vi "Filter and Data Scaling backup (62611) temp.vi"(0 "Offset Data":string[](array[string]), 5 "Slope Data":string[](array[string]), 7 "Filter Data":string[](array[string]), 9 "Vin":dbl[](array[numeric]), 11 "error in":errorcluster, 12 "Allow Zero?":string[](array[string])) -> (4 "Vout":string[](array[string]), 6 "Offset Data":string[](array[string]), 8 "ScaledOut":string[](array[string]), 10 "ScaledOut":dbl[](array[numeric]), 14 "Allow Zero?":string[](array[string]), 15 "error out":errorcluster)   [LabVIEW 2018]
uses:
  Counters.vi
  <vilib>/ptbypt/NI_PtbyPt.lvlib
panel:
  out "k":dbl
  out "fdelta":dbl
  out "fratio":dbl
  out "dp":dbl
  out "Numeric":i32
  # "32-51= FM1 GPM Data Point 1-20"
  # "32-51= FM1 Data Point # 1-20"
  # "32-51 = FM1 K Factor 1-20"
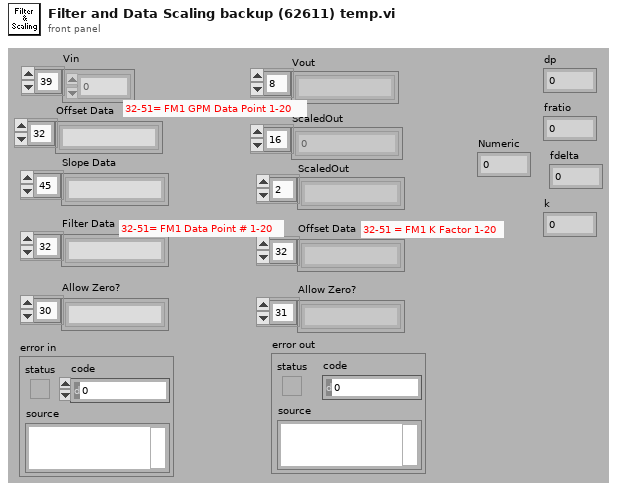
[diagram p1: front panel]
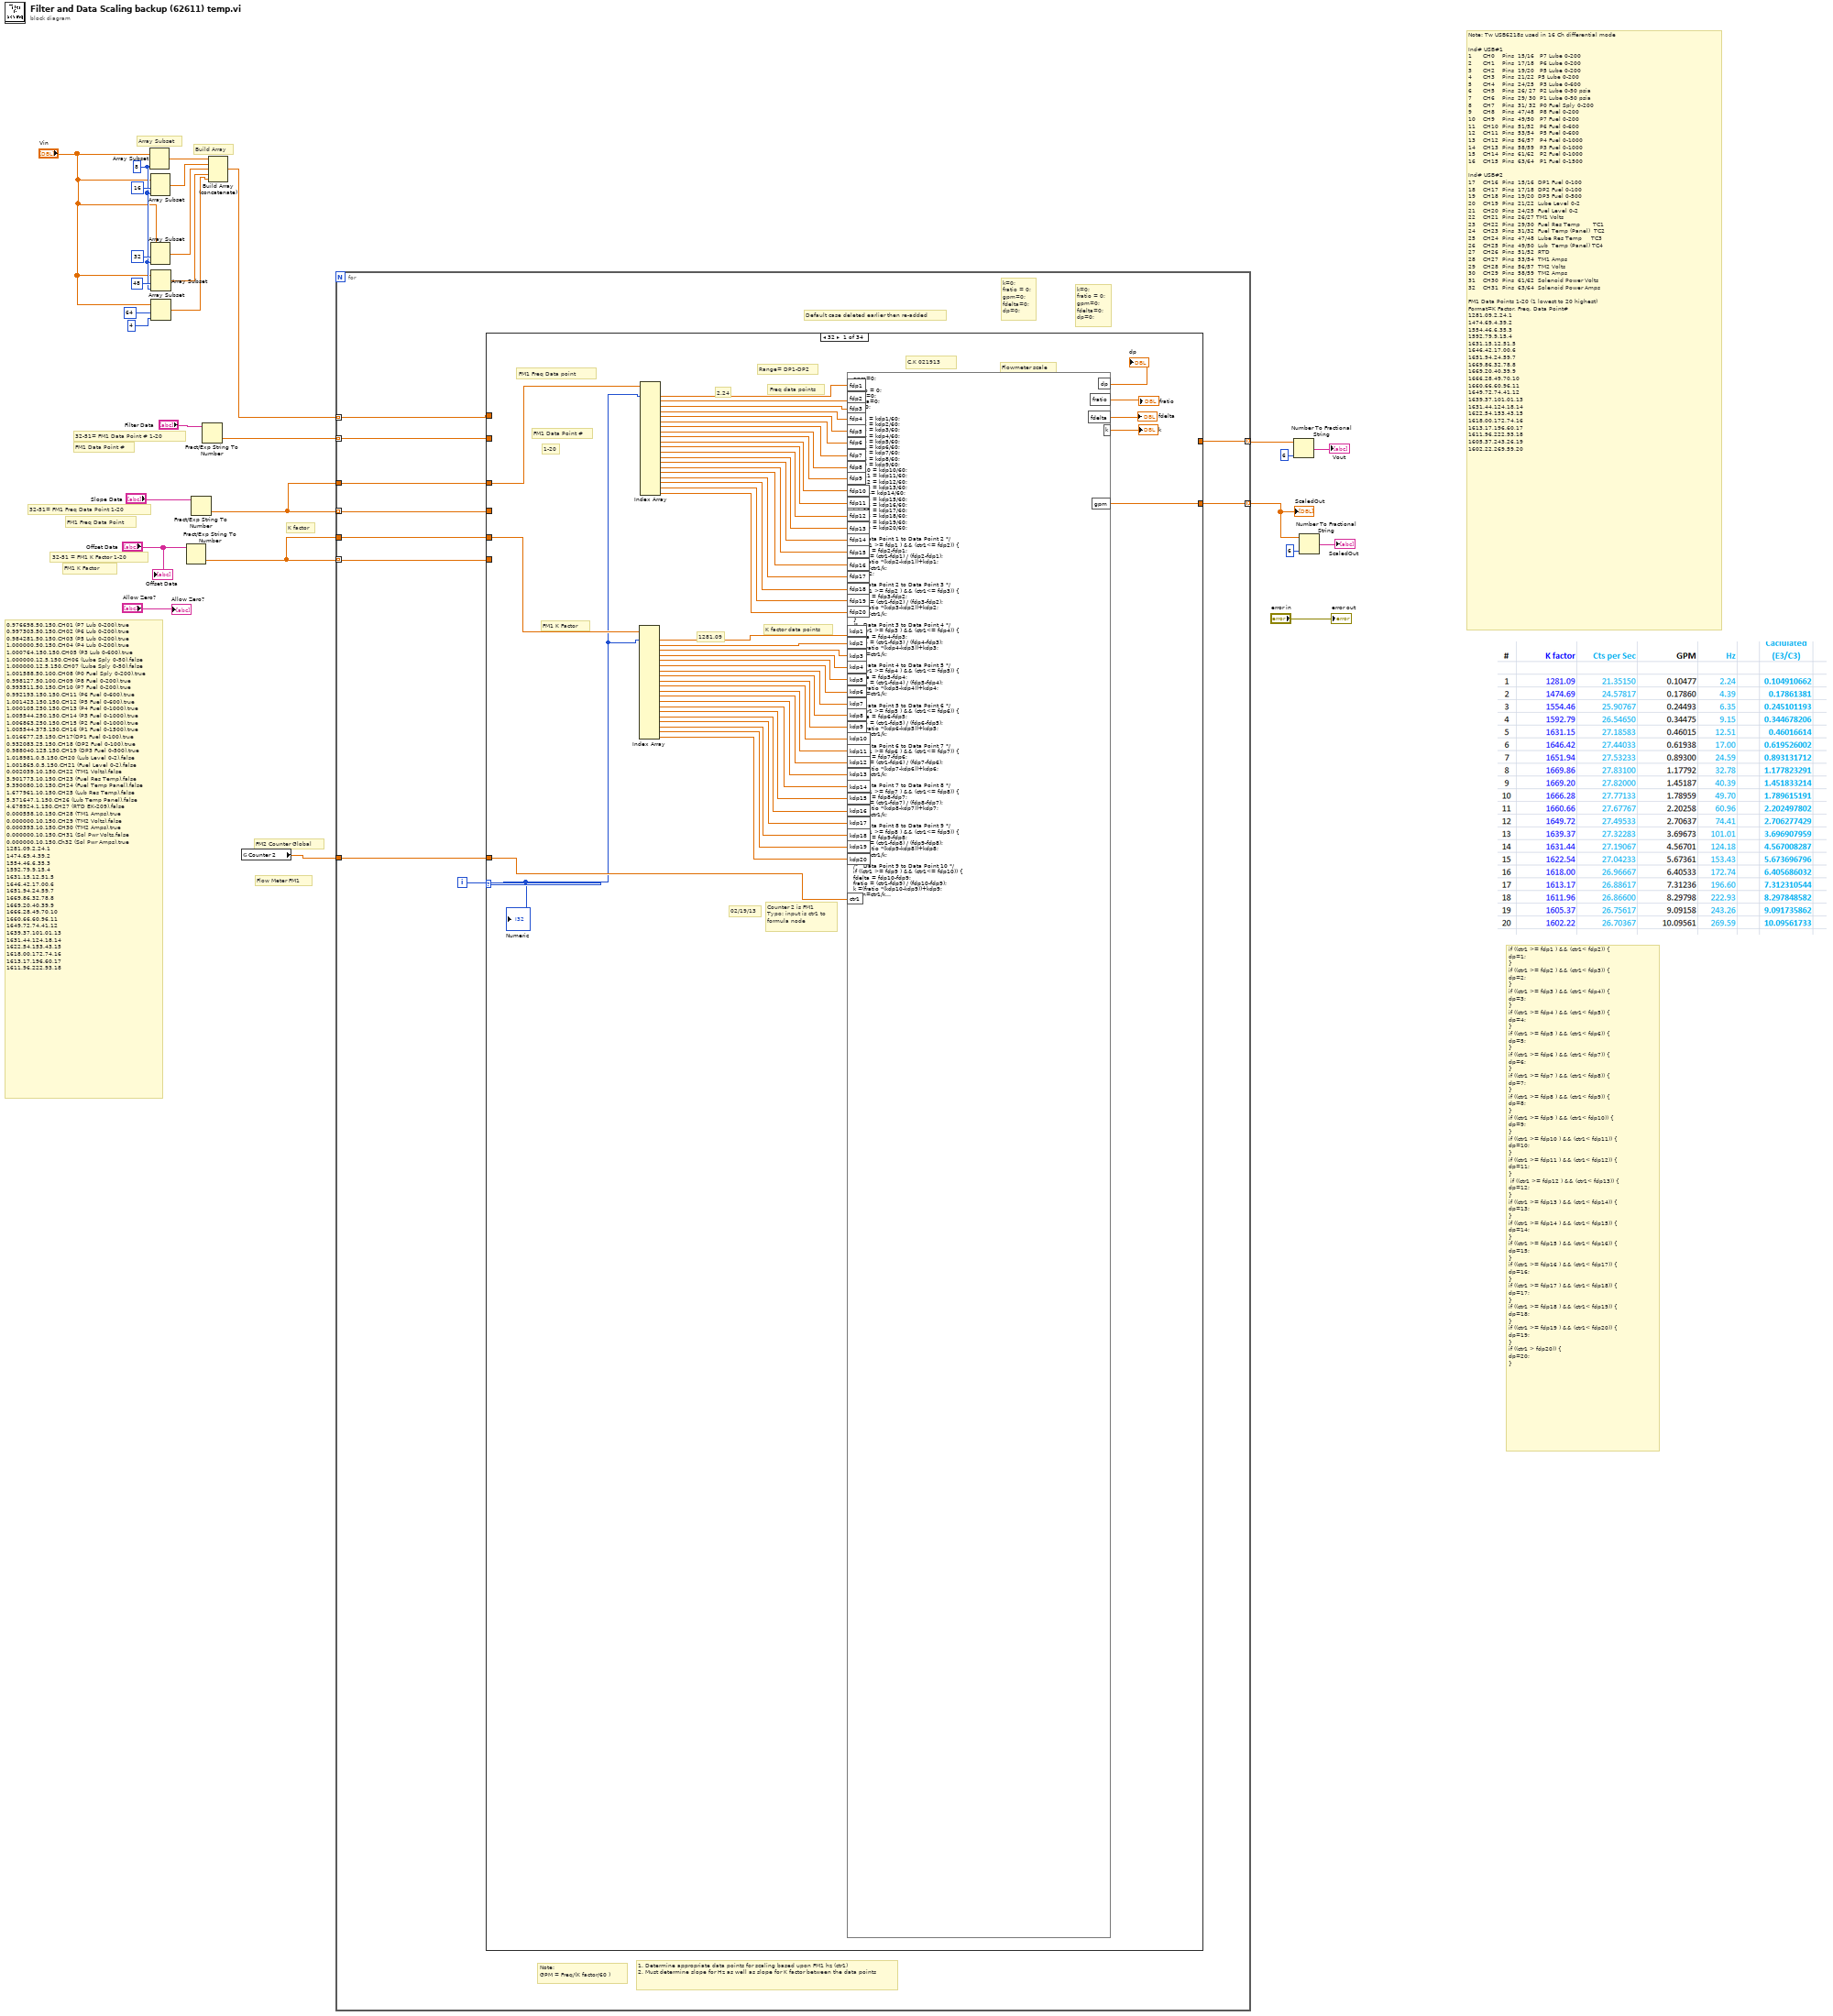
[diagram p0: block diagram]
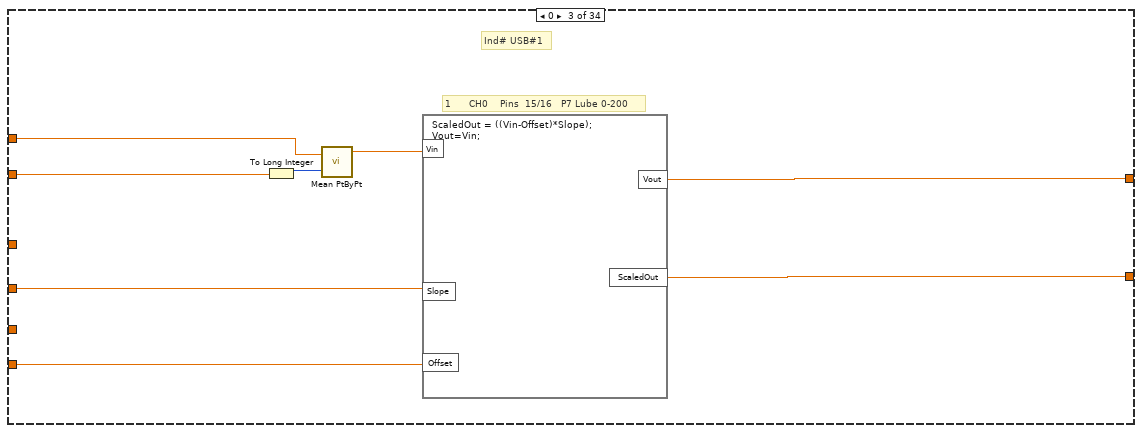
[diagram p3: hidden frame]
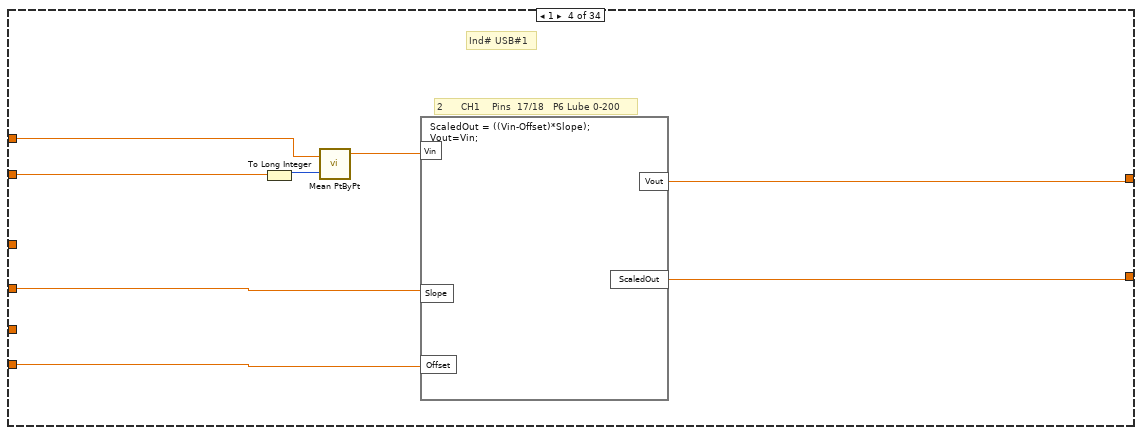
[diagram p4: hidden frame]
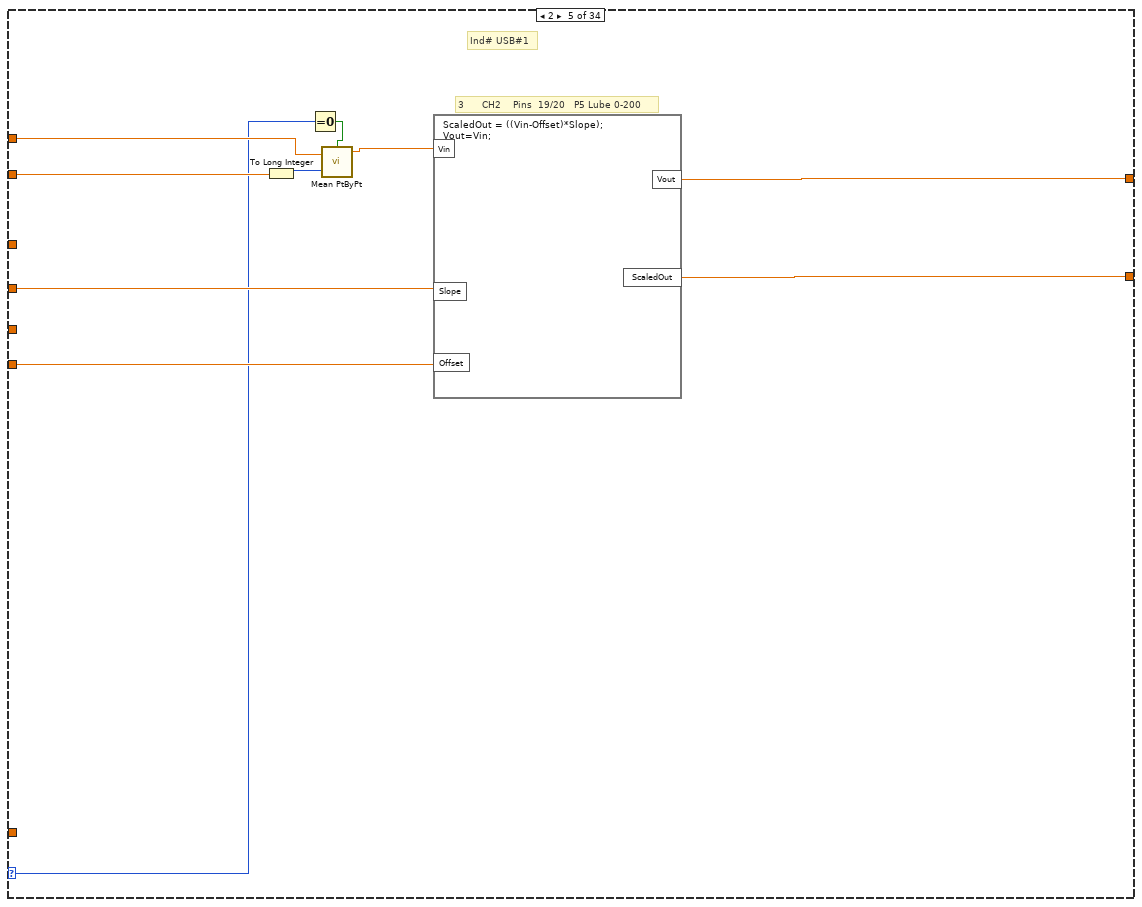
[diagram p5: hidden frame]
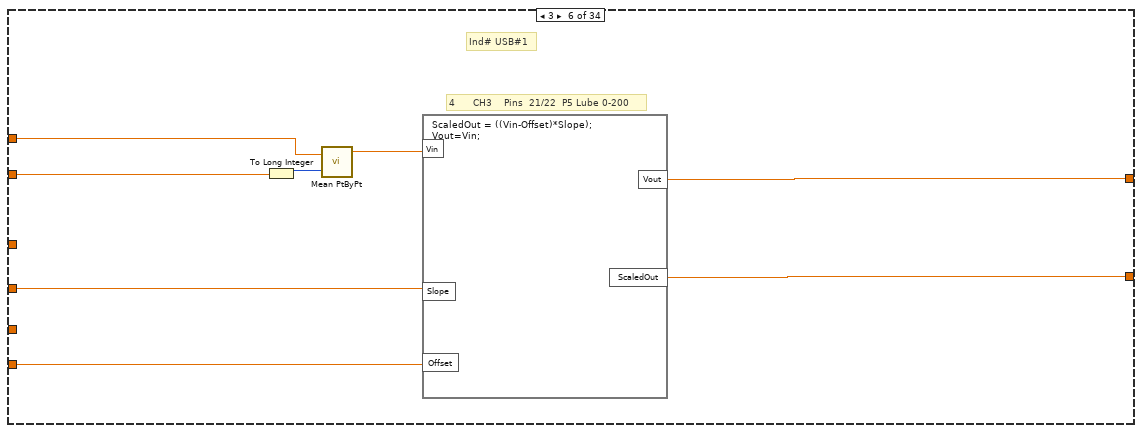
[diagram p6: hidden frame]
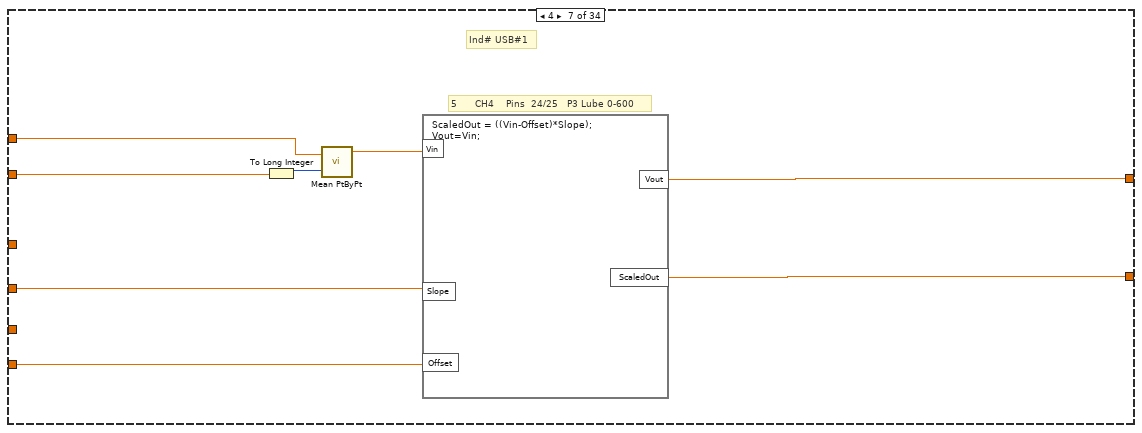
[diagram p7: hidden frame]
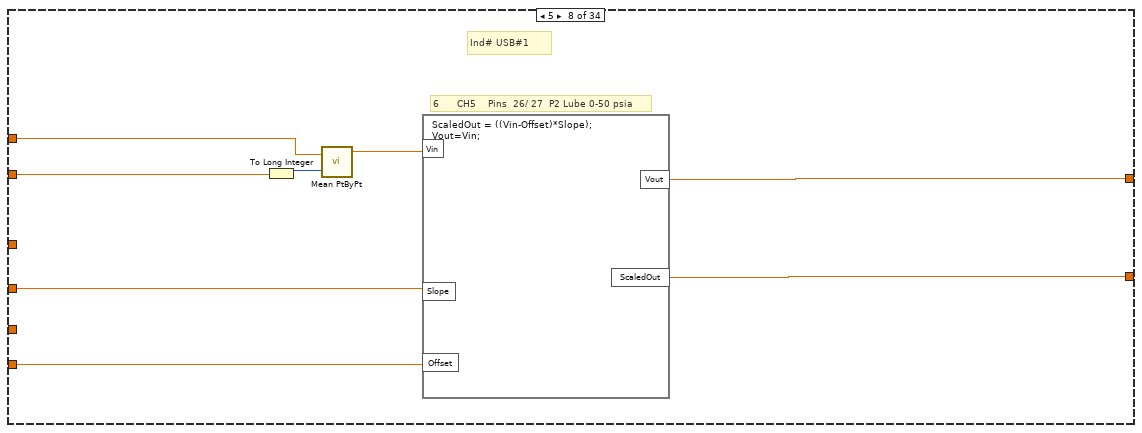
[diagram p8: hidden frame]
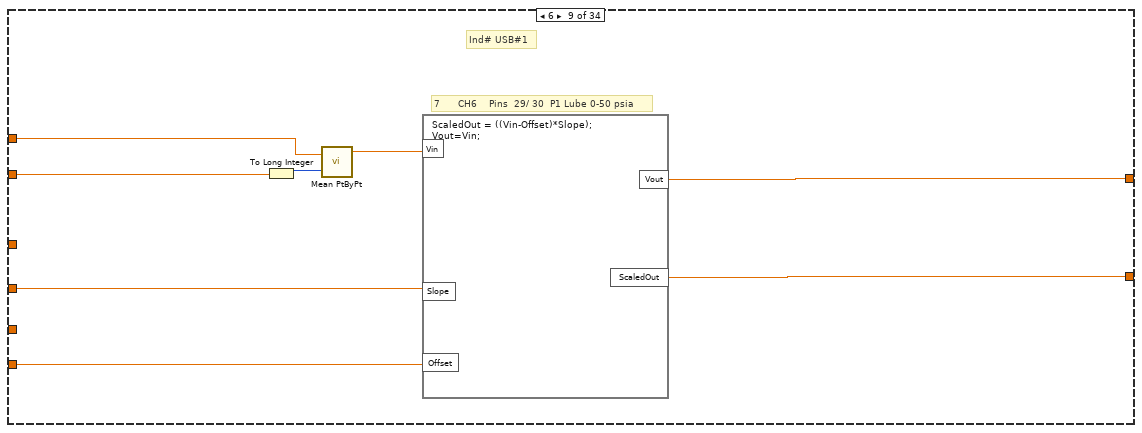
[diagram p9: hidden frame]
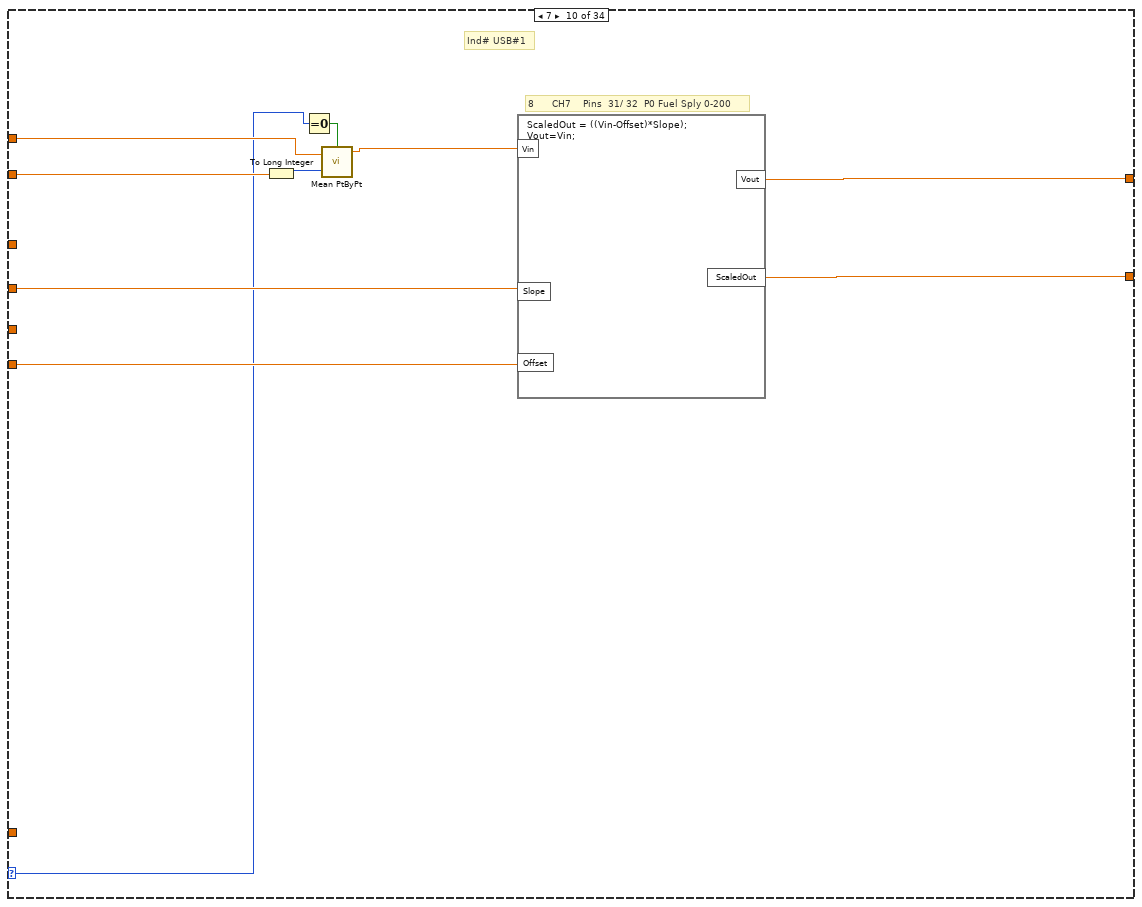
[diagram p10: hidden frame]
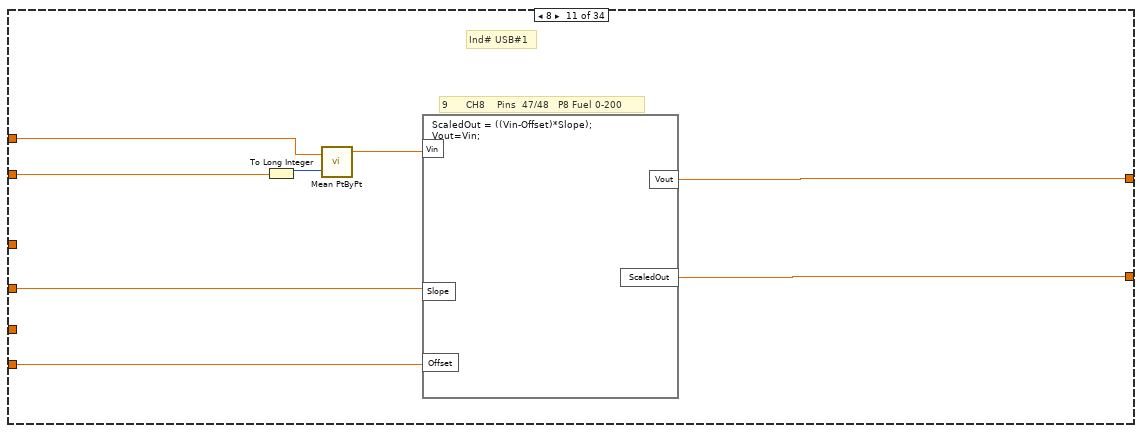
[diagram p11: hidden frame]
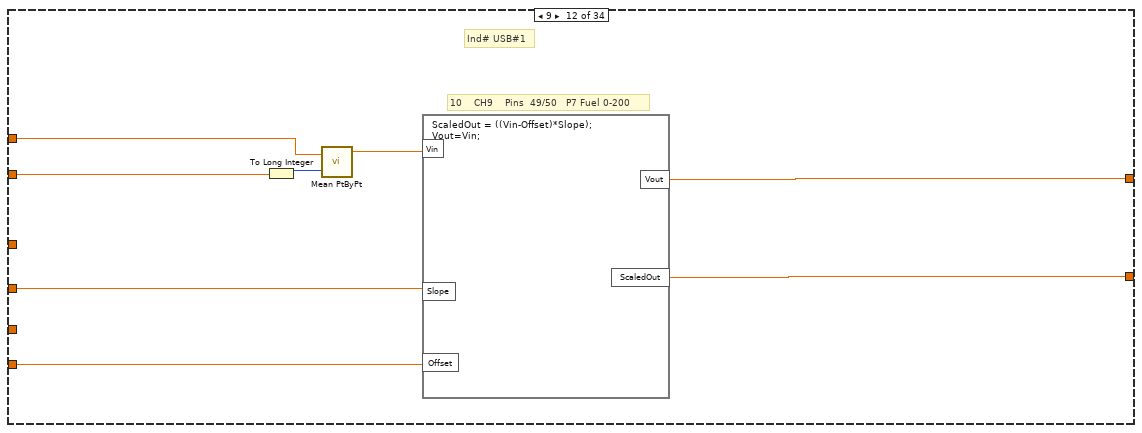
[diagram p12: hidden frame]
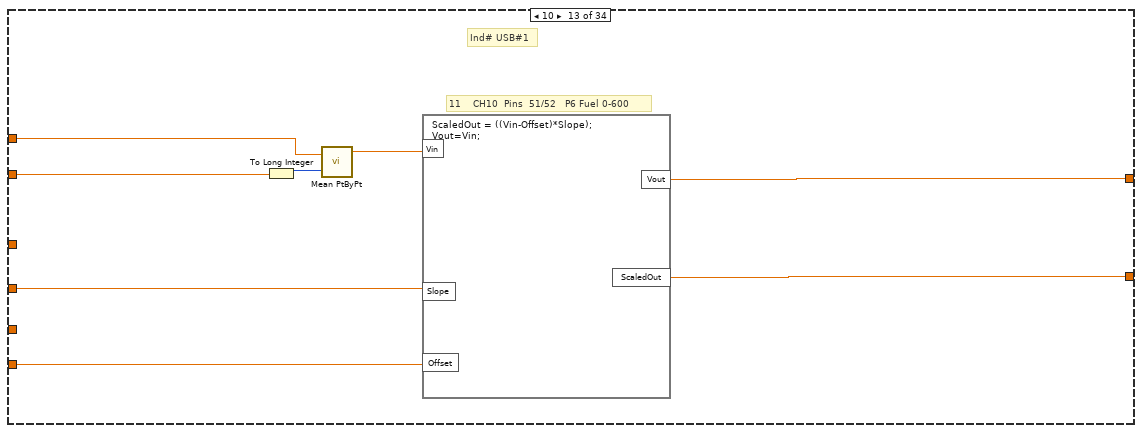
[diagram p13: hidden frame]
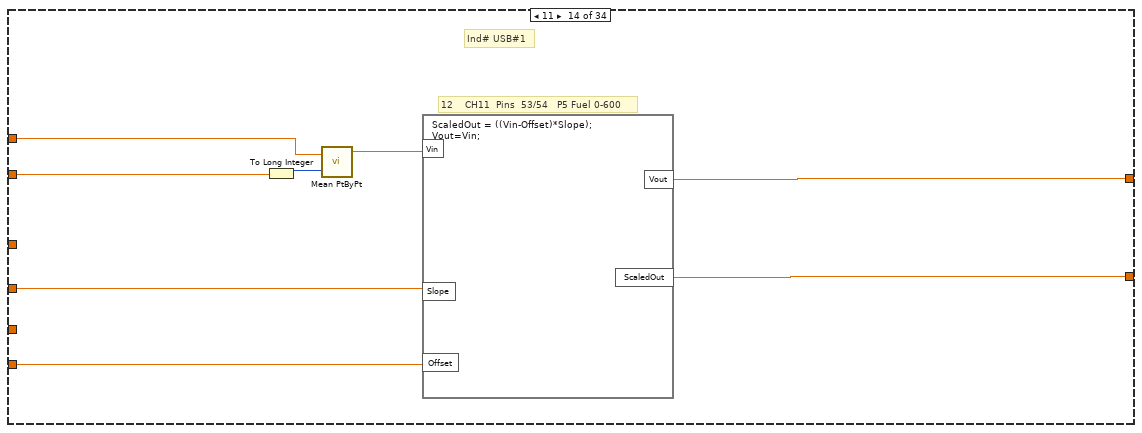
[diagram p14: hidden frame]
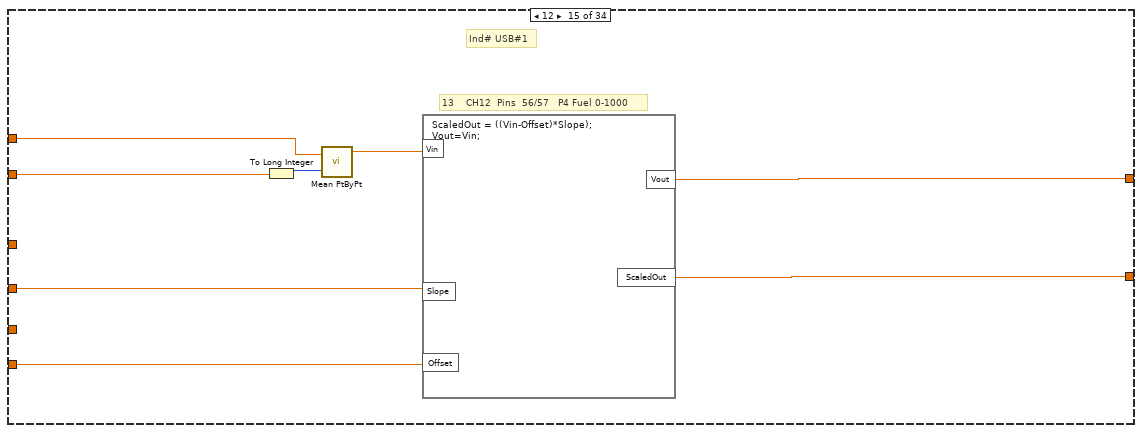
[diagram p15: hidden frame]
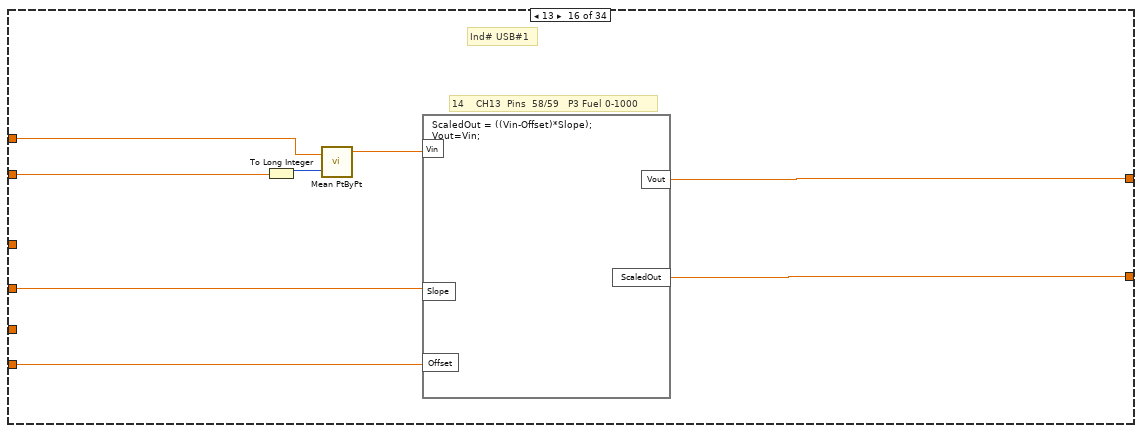
[diagram p16: hidden frame]
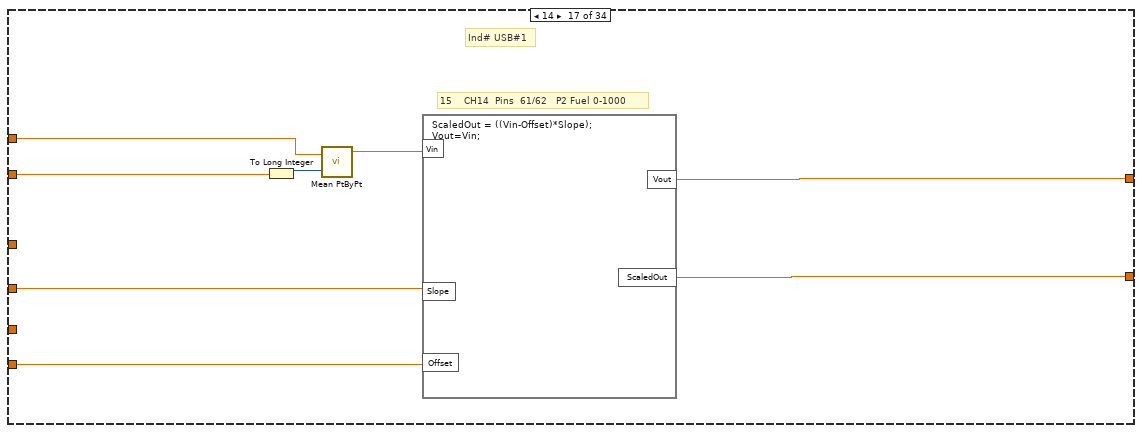
[diagram p17: hidden frame]
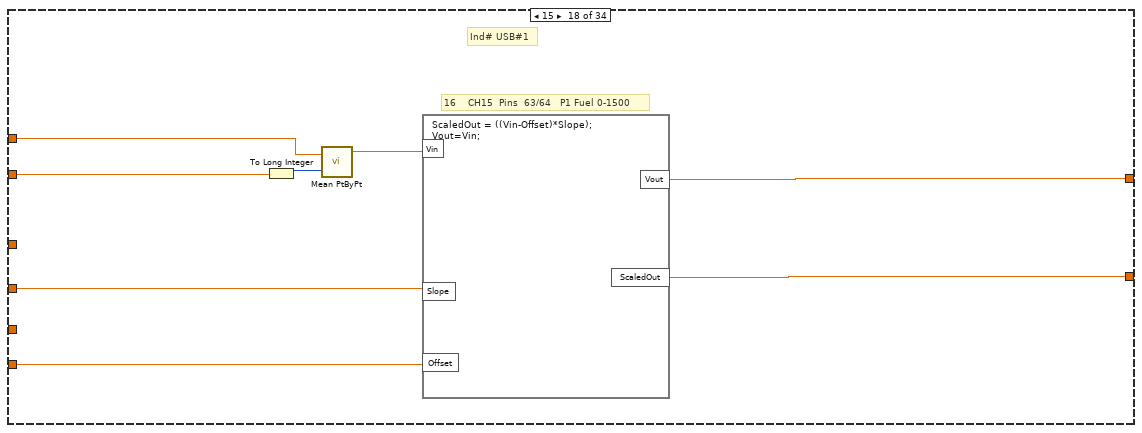
[diagram p18: hidden frame]
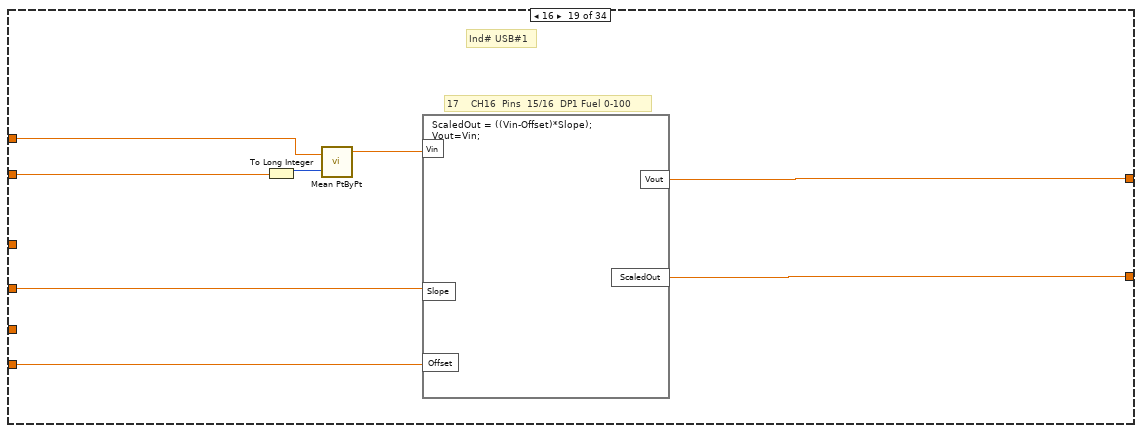
[diagram p19: hidden frame]
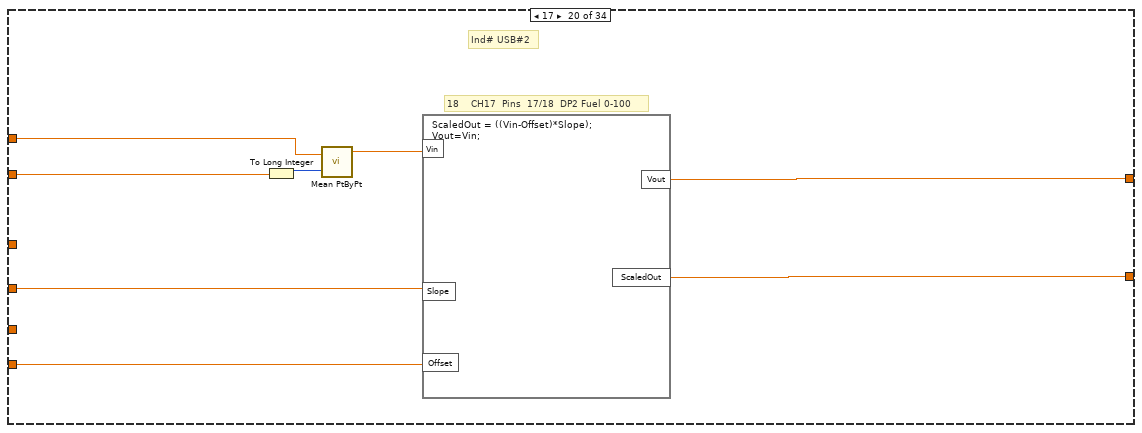
[diagram p20: hidden frame]
diagram:
  w11 = 8 ("length")
  # "0.976698,50,150,CH01 (P7 Lub 0-200),true\n0.997303,50,150,CH02 (P6 Lub 0-200),true\n0.984281,50,150,CH03 (P5 Lub 0-200),true\n1.000000,50,150,CH04 (P4 Lub 0-200),true\n1.000764,150,150,CH05 (P3 Lub 0-600),true\n1.000000,12.5,150,CH06 (Lube Sply 0-50),false\n1.000000,12.5,150,CH07 (Lube Sply 0-50),false\n1.001588,50,100,CH08 (P0 Fuel Sply 0-200),true\n0.998127,50,100,CH09 (P8 Fuel 0-200),true\n0.993511,50,150,CH10 (P7 Fuel 0-200),true\n0.992193,150,150,CH11 (P6 Fuel 0-600),true\n1.001423,150,150,CH12 (P5 Fuel 0-600),true\n1.000105,250,150,CH13 (P4 Fuel 0-1000),true\n1.005544,250,150,CH14 (P3 Fuel 0-1000),true\n1.006863,250,150,CH15 (P2 Fuel 0-1000),true\n1.005544,375,150,CH16 (P1 Fuel 0-1500),true\n1.016677,25,150,CH17(DP1 Fuel 0-100),true\n0.932083,25,150,CH18 (DP2 Fuel 0-100),true\n0.988040,125,150,CH19 (DP3 Fuel 0-500),true\n1.018981,0.5,150,CH20 (Lub Level 0-2),false\n1.001865,0.5,150,CH21 (Fuel Level 0-2),false\n0.002039,10,150,CH22 (TM1 Volts),false\n3.901773,10,150,CH23 (Fuel Res Temp),false\n5.390080,10,150,CH24 (Fuel Temp Panel),false\n1.677961,10,150,CH25 (Lub Res Temp),false\n5.371647,1,150,CH26 (Lub Temp Panel),false\n4.678924,1,150,CH27 (RTD EK-209),false\n0.000558,10,150,CH28 (TM1 Amps),true\n0.000000,10,150,CH29 (TM2 Volts),false\n0.000393,10,150,CH30 (TM2 Amps),true\n0.000000,10,150,CH31 (Sol Pwr Volts,false\n0.000000,10,150,Ch32 (Sol Pwr Amps),true\n1281.09,2.24,1\n1474.69,4.39,2\n1554.46,6.35,3\n1592.79,9.15,4\n1631.15,12.51,5\n1646.42,17.00,6\n1651.94,24.59,7\n1669.86,32.78,8\n1669.20,40.39,9\n1666.28,49.70,10\n1660.66,60.96,11\n1649.72,74.41,12\n1639.37,101.01,13\n1631.44,124.18,14\n1622.54,153.43,15\n1618.00,172.74,16\n1613.17,196.60,17\n1611.96,222.93,18"
  # "Flow Meter FM1"
  # "if ((ctr1 >= fdp1 ) && (ctr1< fdp2)) {\ndp=1;\n}\nif ((ctr1 >= fdp2 ) && (ctr1< fdp3)) {\ndp=2;\n}\nif ((ctr1 >= fdp3 ) && (ctr1< fdp4)) {\ndp=3;\n}\nif ((ctr1 >= fdp4 ) && (ctr1< fdp5)) {\ndp=4;\n}\nif ((ctr1 >= fdp5 ) && (ctr1< fdp6)) {\ndp=5;\n}\nif ((ctr1 >= fdp6 ) && (ctr1< fdp7)) {\ndp=6;\n}\nif ((ctr1 >= fdp7 ) && (ctr1< fdp8)) {\ndp=7;\n}\nif ((ctr1 >= fdp8 ) && (ctr1< fdp9)) {\ndp=8;\n}\nif ((ctr1 >= fdp9 ) && (ctr1< fdp10)) {\ndp=9;\n}\nif ((ctr1 >= fdp10 ) && (ctr1< fdp11)) {\ndp=10;\n}\nif ((ctr1 >= fdp11 ) && (ctr1< fdp12)) {\ndp=11;\n}\n if ((ctr1 >= fdp12 ) && (ctr1< fdp13)) {\ndp=12;\n}\nif ((ctr1 >= fdp13 ) && (ctr1< fdp14)) {\ndp=13;\n}\nif ((ctr1 >= fdp14 ) && (ctr1< fdp15)) {\ndp=14;\n}\nif ((ctr1 >= fdp15 ) && (ctr1< fdp16)) {\ndp=15;\n}\nif ((ctr1 >= fdp16 ) && (ctr1< fdp17)) {\ndp=16;\n}\nif ((ctr1 >= fdp17 ) && (ctr1< fdp18)) {\ndp=17;\n}\nif ((ctr1 >= fdp18 ) && (ctr1< fdp19)) {\ndp=18;\n}\nif ((ctr1 >= fdp19 ) && (ctr1< fdp20)) {\ndp=19;\n}\nif ((ctr1 > fdp20)) {\ndp=20;\n}"
  # "Note: Tw USB6218s used in 16 Ch differential mode\n\nInd# USB#1\n1      CH0\t\t  Pins  15/16\t  P7 Lube 0-200\n2      CH1\t\t  Pins  17/18\t  P6 Lube 0-200\n3      CH2\t\t  Pins  19/20   P5 Lube 0-200\n4      CH3\t\t  Pins  21/22  P5 Lube 0-200\n5      CH4\t   Pins  24/25\t  P3 Lube 0-600\n6      CH5\t\t  Pins  26/\t27\t P2 Lube 0-50 psia\n7      CH6\t   Pins  29/\t30\t P1 Lube 0-50 psia\n8      CH7\t  \tPins  31/ 32\t P0 Fuel Sply 0-200  \n9      CH8\t  \tPins  47/48\t  P8 Fuel 0-200   \n10    CH9\t\t  Pins  49/50\t  P7 Fuel 0-200   \n11    CH10\t\tPins  51/52\t  P6 Fuel 0-600   \n12    CH11\t\tPins  53/54\t  P5 Fuel 0-600   \n13    CH12\t\tPins  56/57\t  P4 Fuel 0-1000 \n14    CH13\t\tPins  58/59\t  P3 Fuel 0-1000 \n15    CH14\t\tPins  61/62 \t P2 Fuel 0-1000  \n16    CH15\t\tPins  63/64 \t P1 Fuel 0-1500 \n\nInd# USB#2\n17    CH16\t\tPins  15/16\t DP1 Fuel 0-100 \n18    CH17\t\tPins  17/18\t DP2 Fuel 0-100\n19    CH18\t\tPins  19/20  DP3 Fuel 0-500 \n20    CH19\t Pins  21/22\t Lube Level 0-2 \n21    CH20\t\tPins  24/25\t Fuel Level 0-2 \n22    CH21\t\tPins  26/27\tTM1 Volts  \n23    CH22\t Pins  29/30  Fuel Res Temp       TC1\n24    CH23\t\tPins  31/32\t Fuel Temp (Panel)  TC2 \n25    CH24\t\tPins \t47/48\t Lube Res Temp     TC3 \n26    CH25\t\tPins  49/50\t Lub  Temp (Panel) TC4 \n27    CH26\t\tPins  51/52\t RTD \n28    CH27\t\tPins  53/54\t TM1 Amps \n29    CH28\t\tPins  56/57\t TM2 Volts\n30    CH29\t\tPins  58/59\t TM2 Amps \n31    CH30\t\tPins  61/62  Solenoid Power Volts \n32    CH31\t\tPins  63/64  Solenoid Power Amps\n\nFM1 Data Points 1-20 (1 lowest to 20 highest)\nFormat=K Factor, Freq, Data Point#\n1281.09,2.24,1\n1474.69,4.39,2\n1554.46,6.35,3\n1592.79,9.15,4\n1631.15,12.51,5\n1646.42,17.00,6\n1651.94,24.59,7\n1669.86,32.78,8\n1669.20,40.39,9\n1666.28,49.70,10\n1660.66,60.96,11\n1649.72,74.41,12\n1639.37,101.01,13\n1631.44,124.18,14\n1622.54,153.43,15\n1618.00,172.74,16\n1613.17,196.60,17\n1611.96,222.93,18\n1605.37,243.26,19\n1602.22,269.59,20"
  # "K factor"
  # "FM1 Freq Data Point"
  # "FM2 Counter Global"
  # "FM1 Data Point #"
  # "FM1 K Factor"
  # "32-51 = FM1 K Factor 1-20"
  # "32-51= FM1 Data Point # 1-20"
  # "32-51= FM1 Freq Data Point 1-20"
  # "Array Subset"
  # "Build Array"
  n1 = Array Subset(array="Vin", length=w11) -> (w16:dbl[])  [unwired: 1 in]
  n2 = Array Subset(array="Vin", index=16, length=w11) -> (w15:dbl[])
  n3 = Array Subset(array="Vin", index=32, length=w11) -> (w13:dbl[])
  n4 = Array Subset(array="Vin", index=48, length=w11) -> (w14:dbl[])
  n5 = Array Subset(array="Vin", index=64, length=4 ("index")) -> (w6:dbl[])
  n6 = Fract/Exp String To Number(string="Offset Data") -> (number=w3:dbl[])  [unwired: 4 out]
  n7 = Fract/Exp String To Number(string="Slope Data") -> (number=w4:dbl[])  [unwired: 4 out]
  n8 = Fract/Exp String To Number(string="Filter Data") -> (number=w2:dbl[])  [unwired: 4 out]
  n9 = Build Array (concatenate)(w16, w15, w13, w14, w6) -> (w5:dbl[])
  n10 = global read "Counters.vi" "Counter 2"() -> (w1:dbl)
  n11 = for {
    tunnel: w4 -> [w37] mode=indexing
    tunnel: w3 -> [w32] mode=indexing
    tunnel: w2 -> [w38] mode=indexing
    tunnel: [w35] -> w10 mode=indexing
    tunnel: [w36] -> w19 mode=indexing
    tunnel: w5 -> [w33] mode=indexing
    tunnel: w4 -> [w31]
    tunnel: w3 -> [w30]
    tunnel: w1 -> [w29]
    i -> [w34]
    # "k=0;\nfratio = 0;\ngpm=0;\nfdelta=0;\ndp=0;"
    # "k=0;\nfratio = 0;\ngpm=0;\nfdelta=0;\ndp=0;"
    # "Note:\nGPM = Freq/(K factor/60 )"
    # "1. Determine appropriate data points for scaling based upon FM1 hz (ctr1)\n2. Must determine slope for Hz as well as slope for K factor between the data points"
    # "Default case deleted earlier then re-added"
    n12 = case shown="32" w34 {
      selector: w34 -> [w39 _ _ _ w107 _ _ _ _ w149 _ _ _ _ _ _ _ _ _ _ _ _ _ _ _ _ _ _ _ _ _ _ _ _]
      tunnel: w33 -> [_ _ w92 w98 w112 w118 w126 w134 w142 w154 w160 w168 w176 w184 w192 w200 w208 w216 w224 w232 w240 w248 w256 w264 w272 w280 w288 w296 w304 w312 w320 w328 w336 w344]
      tunnel: w38 -> [_ _ w93 w99 w113 w119 w127 w135 w143 w155 w161 w169 w177 w185 w193 w201 w209 w217 w225 w233 w241 w249 w257 w265 w273 w281 w289 w297 w305 w313 w321 w329 w337 w345]
      tunnel: w37 -> [_ _ w91 w101 w111 w117 w125 w133 w141 w153 w159 w167 w175 w183 w191 w199 w207 w215 w223 w231 w239 w247 w255 w263 w271 w279 w287 w295 w303 w311 w319 w327 w335 w343]
      tunnel: w32 -> [_ _ w90 w100 w110 w116 w124 w132 w140 w152 w158 w166 w174 w182 w190 w198 w206 w214 w222 w230 w238 w246 w254 w262 w270 w278 w286 w294 w302 w310 w318 w326 w334 w342]
      tunnel: [_ _ w88 w97 w108 w114 w122 w130 w138 w150 w156 w164 w172 w180 w188 w196 w204 w212 w220 w228 w236 w244 w252 w261 w268 w276 w284 w292 w300 w309 w317 w325 w333 w341] -> w36
      tunnel: [w44 _ w89 w96 w109 w115 w123 w131 w139 w151 w157 w165 w173 w181 w189 w197 w205 w213 w221 w229 w237 w245 w253 w260 w269 w277 w285 w293 w301 w308 w316 w324 w332 w340] -> w35
      tunnel: w31 -> [w86 _ _ _ _ _ _ _ _ _ _ _ _ _ _ _ _ _ _ _ _ _ _ _ _ _ _ _ _ _ _ _ _ _]
      tunnel: w30 -> [w85 _ _ _ _ _ _ _ _ _ _ _ _ _ _ _ _ _ _ _ _ _ _ _ _ _ _ _ _ _ _ _ _ _]
      tunnel: w29 -> [w87 _ _ _ _ _ _ _ _ _ _ _ _ _ _ _ _ _ _ _ _ _ _ _ _ _ _ _ _ _ _ _ _ _]
      frame 32 {
        # "1281.09"
        # "02/19/13"
        # "Counter 2 is FM1\nTypo: input is ctr1 to\nformula node"
        # "C.K 021913"
        # "2.24"
        # "Range= DP1-DP2"
        # "K factor data points"
        # "Freq data points"
        # "Flowmeter scale"
        # "1-20"
        # "FM1 Data Point #"
        # "FM1 K Factor"
        # "FM1 Freq Data point"
        n13 = Index Array "Index Array"(array=w85, index #1=w39) -> (element #1=w64:dbl, element #2=w63:dbl, element #3=w62:dbl, element #4=w61:dbl, element #5=w60:dbl, element #6=w59:dbl, element #7=w58:dbl, element #8=w57:dbl, element #9=w56:dbl, element #10=w55:dbl, element #11=w54:dbl, element #12=w53:dbl, element #13=w52:dbl, element #14=w51:dbl, element #15=w50:dbl, element #16=w49:dbl, element #17=w48:dbl, element #18=w47:dbl, element #19=w46:dbl, element #20=w45:dbl)  [unwired: 19 in]
        n14 = Index Array "Index Array"(array=w86, index #1=w39) -> (element #1=w84:dbl, element #2=w83:dbl, element #3=w82:dbl, element #4=w81:dbl, element #5=w80:dbl, element #6=w79:dbl, element #7=w78:dbl, element #8=w77:dbl, element #9=w76:dbl, element #10=w75:dbl, element #11=w74:dbl, element #12=w73:dbl, element #13=w72:dbl, element #14=w71:dbl, element #15=w70:dbl, element #16=w69:dbl, element #17=w68:dbl, element #18=w67:dbl, element #19=w66:dbl, element #20=w65:dbl)  [unwired: 19 in]
        n15 = formula code="gpm=0;\nk=0;\nfratio = 0;\ngpm=0;\nfdelta=0;\ndp=0;\n\nkdp1 = kdp1/60;\nkdp2 = kdp2/60;\nkdp3 = kdp3/60;\nkdp4 = kdp4/60;\nkdp5 = kdp5/60;\nkdp6 = kdp6/60;\nkdp7 = kdp7/60;\nkdp8 = kdp8/60;\nkdp9 = kdp9/60;\nkdp10 = kdp10/60;\nkdp11 = kdp11/60;\nkdp12 = kdp12/60;\nkdp13 = kdp13/60;\nkdp14= kdp14/60;\nkdp15 = kdp15/60;\nkdp16 = kdp16/60;\nkdp17 = kdp17/60;\nkdp18 = kdp18/60;\nkdp19 = kdp19/60;\nkdp20 = kdp20/60;\n\n/*   Data Point 1 to Data Point 2 */\nif ((ctr1 >= fdp1 ) && (ctr1<= fdp2)) {\nfdelta = fdp2-fdp1;\nfratio = (ctr1-fdp1) / (fdp2-fdp1);\nk =(fratio *(kdp2-kdp1))+kdp1;\ngpm=ctr1/k;\ndp=12;\n}\n/*   Data Point 2 to Data Point 3 */\nif ((ctr1 >= fdp2 ) && (ctr1<= fdp3)) {\nfdelta = fdp3-fdp2;\nfratio = (ctr1-fdp2) / (fdp3-fdp2);\nk =(fratio *(kdp3-kdp2))+kdp2;\ngpm=ctr1/k;\n}\n/*   Data Point 3 to Data Point 4 */\nif ((ctr1 >= fdp3 ) && (ctr1<= fdp4)) {\nfdelta = fdp4-fdp3;\nfratio = (ctr1-fdp3) / (fdp4-fdp3);\nk =(fratio *(kdp4-kdp3))+kdp3;\ngpm=ctr1/k;\n}\n/*   Data Point 4 to Data Point 5 */\nif ((ctr1 >= fdp4 ) && (ctr1<= fdp5)) {\nfdelta = fdp5-fdp4;\nfratio = (ctr1-fdp4) / (fdp5-fdp4);\nk =(fratio *(kdp5-kdp4))+kdp4;\ngpm=ctr1/k;\n}\n/*   Data Point 5 to Data Point 6 */\nif ((ctr1 >= fdp5 ) && (ctr1<= fdp6)) {\nfdelta = fdp6-fdp5;\nfratio = (ctr1-fdp5) / (fdp6-fdp5);\nk =(fratio *(kdp6-kdp5))+kdp5;\ngpm=ctr1/k;\n}\n/*   Data Point 6 to Data Point 7 */\nif ((ctr1 >= fdp6 ) && (ctr1<= fdp7)) {\nfdelta = fdp7-fdp6;\nfratio = (ctr1-fdp6) / (fdp7-fdp6);\nk =(fratio *(kdp7-kdp6))+kdp6;\ngpm=ctr1/k;\n}\n/*   Data Point 7 to Data Point 8 */\nif ((ctr1 >= fdp7 ) && (ctr1<= fdp8)) {\nfdelta = fdp8-fdp7;\nfratio = (ctr1-fdp7) / (fdp8-fdp7);\nk =(fratio *(kdp8-kdp7))+kdp7;\ngpm=ctr1/k;\n}\n/*   Data Point 8 to Data Point 9 */\nif ((ctr1 >= fdp8 ) && (ctr1<= fdp9)) {\nfdelta = fdp9-fdp8;\nfratio = (ctr1-fdp8) / (fdp9-fdp8);\nk =(fratio *(kdp9-kdp8))+kdp8;\ngpm=ctr1/k;\n}\n/*   Data Point 9 to Data Point 10 */\nif ((ctr1 >= fdp9 ) && (ctr1<= fdp10)) {\nfdelta = fdp10-fdp9;\nfratio = (ctr1-fdp9) / (fdp10-fdp9);\nk =(fratio *(kdp10-kdp9))+kdp9;\ngpm=ctr1/k;\n}\n/*   Data Point 10 to Data Point 11 */\nif ((ctr1 >= fdp10 ) && (ctr1<= fdp11)) {\nfdelta = fdp11-fdp10;\nfratio = (ctr1-fdp10) / (fdp11-fdp10);\nk =(fratio *(kdp11-kdp10))+kdp10;\ngpm=ctr1/k;\n}\n/*   Data Point 11 to Data Point 12 */\nif ((ctr1 >= fdp11 ) && (ctr1<= fdp12)) {\nfdelta = fdp12-fdp11;\nfratio = (ctr1-fdp11) / (fdp12-fdp11);\nk =(fratio *(kdp12-kdp11))+kdp11;\ngpm=ctr1/k;\n}\n/*   Data Point 12 to Data Point 13 */\nif ((ctr1 >= fdp12) && (ctr1<= fdp13)) {\nfdelta = fdp13-fdp12;\nfratio = (ctr1-fdp12) / (fdp13-fdp12);\nk =(fratio *(kdp13-kdp12))+kdp12;\ngpm=ctr1/k;\n}\n/*   Data Point 13 to Data Point 14 */\nif ((ctr1 >= fdp13 ) && (ctr1<= fdp14)) {\nfdelta = fdp14-fdp13;\nfratio = (ctr1-fdp13) / (fdp14-fdp13);\nk =(fratio *(kdp14-kdp13))+kdp13;\ngpm=ctr1/k;\n}\nif ((ctr1 >= fdp14 ) && (ctr1<= fdp15)) {\nfdelta = fdp15-fdp14;\nfratio = (ctr1-fdp14) / (fdp15-fdp14);\nk =(fratio *(kdp15-kdp14))+kdp14;\ngpm=ctr1/k;\n}\n/*   Data Point 15 to Data Point 16 */\nif ((ctr1 >= fdp15 ) && (ctr1<= fdp16)) {\nfdelta = fdp16-fdp15;\nfratio = (ctr1-fdp15) / (fdp16-fdp15);\nk =(fratio *(kdp16-kdp15))+kdp15;\ngpm=ctr1/k;\n}\n/*   Data Point 16 to Data Point 17 */\nif ((ctr1 >= fdp16 ) && (ctr1<= fdp17)) {\nfdelta = fdp17-fdp16;\nfratio = (ctr1-fdp16) / (fdp17-fdp16);\nk =(fratio *(kdp17-kdp16))+kdp16;\ngpm=ctr1/k;\n}\n/*   Data Point 17 to Data Point 18 */\nif ((ctr1 >= fdp17 ) && (ctr1<= fdp18)) {\nfdelta = fdp18-fdp17;\nfratio = (ctr1-fdp17) / (fdp18-fdp17);\nk =(fratio *(kdp18-kdp17))+kdp17;\ngpm=ctr1/k;\n}\n/*   Data Point 18 to Data Point 19 */\nif ((ctr1 >= fdp18 ) && (ctr1<= fdp19)) {\nfdelta = fdp19-fdp18;\nfratio = (ctr1-fdp18) / (fdp19-fdp18);\nk =(fratio *(kdp19-kdp18))+kdp18;\ngpm=ctr1/k;\n}\n/*   Data Point 19 to Data Point 20 */\nif ((ctr1 >= fdp19 ) && (ctr1<= fdp20)) {\nfdelta = fdp20-fdp19;\nfratio = (ctr1-fdp19) / (fdp20-fdp19);\nk =(fratio *(kdp20-kdp19))+kdp19;\ngpm=ctr1/k;\n}\nif (ctr1 >= fdp20) {\nfdelta = fdp20-fdp19;\nfratio = (ctr1-fdp19) / (fdp20-fdp19);\nk =(fratio *(kdp20-kdp19))+kdp19;\ngpm=ctr1/k;\ndp=2021;\n}\n\n/*   Data Point 0 to Data Point 1 temporary */\nif (ctr1 <= fdp1 ) {\nfdelta = fdp2-fdp1;\nfratio = (ctr1-fdp1) / (fdp2-fdp1);\nk =(fratio *(kdp2-kdp1))+kdp1;\ngpm=ctr1/k;\ndp=12;\n}"("fdp1"=w84, "fdp2"=w83, "kdp1"=w64, "ctr1"=w87, "kdp2"=w63, "fdp3"=w82, "fdp4"=w81, "fdp5"=w80, "fdp6"=w79, "fdp7"=w78, "fdp8"=w77, "fdp9"=w76, "fdp10"=w75, "fdp11"=w74, "fdp12"=w73, "fdp13"=w72, "fdp14"=w71, "fdp15"=w70, "fdp16"=w69, "fdp17"=w68, "fdp18"=w67, "fdp19"=w66, "fdp20"=w65, "kdp3"=w62, "kdp4"=w61, "kdp5"=w60, "kdp6"=w59, "kdp7"=w58, "kdp8"=w57, "kdp9"=w56, "kdp10"=w55, "kdp11"=w54, "kdp12"=w53, "kdp13"=w52, "kdp14"=w51, "kdp15"=w50, "kdp16"=w49, "kdp17"=w48, "kdp18"=w47, "kdp19"=w46, "kdp20"=w45) -> ("gpm"=w44:dbl, "fratio"=→"fratio":dbl, "fdelta"=→"fdelta":dbl, "k"=→"k":dbl, "dp"=→"dp":dbl)
        "Numeric" <- w39
      }
      frame 33, Default {
      }
      frame 0 {
        # "Ind# USB#1"
        # "1      CH0\t\t  Pins  15/16\t  P7 Lube 0-200"
        n16 = To Long Integer(number=w93) -> (32bit integer=w95:i32)
        n17 = call <vilib>:"Mean PtByPt.vi"("x"=w92, "sample length"=w95) -> ("mean"=w94:dbl)  [unwired: 1 in, 2 out]
        n18 = formula code="ScaledOut = ((Vin-Offset)*Slope);\nVout=Vin;"("Vin"=w94, "Slope"=w91, "Offset"=w90) -> ("ScaledOut"=w89:dbl, "Vout"=w88:dbl)
      }
      frame 1 {
        # "Ind# USB#1"
        # "2      CH1\t\t  Pins  17/18\t  P6 Lube 0-200"
        n19 = To Long Integer(number=w99) -> (32bit integer=w103:i32)
        n20 = call <vilib>:"Mean PtByPt.vi"("x"=w98, "sample length"=w103) -> ("mean"=w102:dbl)  [unwired: 1 in, 2 out]
        n21 = formula code="ScaledOut = ((Vin-Offset)*Slope);\nVout=Vin;"("Vin"=w102, "Slope"=w101, "Offset"=w100) -> ("ScaledOut"=w96:dbl, "Vout"=w97:dbl)
      }
      frame 2 {
        # "Ind# USB#1"
        # "3      CH2\t\t  Pins  19/20   P5 Lube 0-200"
        n22 = To Long Integer(number=w113) -> (32bit integer=w106:i32)
        n23 = Equal To 0?(x=w107) -> (x = 0?=w105:bool)
        n24 = call <vilib>:"Mean PtByPt.vi"("x"=w112, "sample length"=w106, "initialize"=w105) -> ("mean"=w104:dbl)  [unwired: 2 out]
        n25 = formula code="ScaledOut = ((Vin-Offset)*Slope);\nVout=Vin;"("Vin"=w104, "Slope"=w111, "Offset"=w110) -> ("ScaledOut"=w109:dbl, "Vout"=w108:dbl)
      }
      frame 3 {
        # "Ind# USB#1"
        # "4      CH3\t\t  Pins  21/22  P5 Lube 0-200"
        n26 = To Long Integer(number=w119) -> (32bit integer=w121:i32)
        n27 = call <vilib>:"Mean PtByPt.vi"("x"=w118, "sample length"=w121) -> ("mean"=w120:dbl)  [unwired: 1 in, 2 out]
        n28 = formula code="ScaledOut = ((Vin-Offset)*Slope);\nVout=Vin;"("Vin"=w120, "Slope"=w117, "Offset"=w116) -> ("ScaledOut"=w115:dbl, "Vout"=w114:dbl)
      }
      frame 4 {
        # "Ind# USB#1"
        # "5      CH4\t   Pins  24/25\t  P3 Lube 0-600"
        n29 = To Long Integer(number=w127) -> (32bit integer=w129:i32)
        n30 = call <vilib>:"Mean PtByPt.vi"("x"=w126, "sample length"=w129) -> ("mean"=w128:dbl)  [unwired: 1 in, 2 out]
        n31 = formula code="ScaledOut = ((Vin-Offset)*Slope);\nVout=Vin;"("Vin"=w128, "Slope"=w125, "Offset"=w124) -> ("ScaledOut"=w123:dbl, "Vout"=w122:dbl)
      }
      frame 5 {
        # "6      CH5\t\t  Pins  26/\t27\t P2 Lube 0-50 psia"
        # "Ind# USB#1"
        n32 = To Long Integer(number=w135) -> (32bit integer=w137:i32)
        n33 = call <vilib>:"Mean PtByPt.vi"("x"=w134, "sample length"=w137) -> ("mean"=w136:dbl)  [unwired: 1 in, 2 out]
        n34 = formula code="ScaledOut = ((Vin-Offset)*Slope);\nVout=Vin;"("Vin"=w136, "Slope"=w133, "Offset"=w132) -> ("ScaledOut"=w131:dbl, "Vout"=w130:dbl)
      }
      frame 6 {
        # "7      CH6\t   Pins  29/\t30\t P1 Lube 0-50 psia"
        # "Ind# USB#1"
        n35 = To Long Integer(number=w143) -> (32bit integer=w145:i32)
        n36 = call <vilib>:"Mean PtByPt.vi"("x"=w142, "sample length"=w145) -> ("mean"=w144:dbl)  [unwired: 1 in, 2 out]
        n37 = formula code="ScaledOut = ((Vin-Offset)*Slope);\nVout=Vin;"("Vin"=w144, "Slope"=w141, "Offset"=w140) -> ("ScaledOut"=w139:dbl, "Vout"=w138:dbl)
      }
      frame 7 {
        # "8      CH7\t  \tPins  31/ 32\t P0 Fuel Sply 0-200"
        # "Ind# USB#1"
        n38 = To Long Integer(number=w155) -> (32bit integer=w147:i32)
        n39 = Equal To 0?(x=w149) -> (x = 0?=w148:bool)
        n40 = call <vilib>:"Mean PtByPt.vi"("x"=w154, "sample length"=w147, "initialize"=w148) -> ("mean"=w146:dbl)  [unwired: 2 out]
        n41 = formula code="ScaledOut = ((Vin-Offset)*Slope);\nVout=Vin;"("Vin"=w146, "Slope"=w153, "Offset"=w152) -> ("ScaledOut"=w151:dbl, "Vout"=w150:dbl)
      }
      frame 8 {
        # "9      CH8\t  \tPins  47/48\t  P8 Fuel 0-200"
        # "Ind# USB#1"
        n42 = To Long Integer(number=w161) -> (32bit integer=w163:i32)
        n43 = call <vilib>:"Mean PtByPt.vi"("x"=w160, "sample length"=w163) -> ("mean"=w162:dbl)  [unwired: 1 in, 2 out]
        n44 = formula code="ScaledOut = ((Vin-Offset)*Slope);\nVout=Vin;"("Vin"=w162, "Slope"=w159, "Offset"=w158) -> ("ScaledOut"=w157:dbl, "Vout"=w156:dbl)
      }
      frame 9 {
        # "10    CH9\t\t  Pins  49/50\t  P7 Fuel 0-200"
        # "Ind# USB#1"
        n45 = To Long Integer(number=w169) -> (32bit integer=w171:i32)
        n46 = call <vilib>:"Mean PtByPt.vi"("x"=w168, "sample length"=w171) -> ("mean"=w170:dbl)  [unwired: 1 in, 2 out]
        n47 = formula code="ScaledOut = ((Vin-Offset)*Slope);\nVout=Vin;"("Vin"=w170, "Slope"=w167, "Offset"=w166) -> ("ScaledOut"=w165:dbl, "Vout"=w164:dbl)
      }
      frame 10 {
        # "11    CH10\t\tPins  51/52\t  P6 Fuel 0-600"
        # "Ind# USB#1"
        n48 = To Long Integer(number=w177) -> (32bit integer=w179:i32)
        n49 = call <vilib>:"Mean PtByPt.vi"("x"=w176, "sample length"=w179) -> ("mean"=w178:dbl)  [unwired: 1 in, 2 out]
        n50 = formula code="ScaledOut = ((Vin-Offset)*Slope);\nVout=Vin;"("Vin"=w178, "Slope"=w175, "Offset"=w174) -> ("ScaledOut"=w173:dbl, "Vout"=w172:dbl)
      }
      frame 11 {
        # "12    CH11\t\tPins  53/54\t  P5 Fuel 0-600"
        # "Ind# USB#1"
        n51 = To Long Integer(number=w185) -> (32bit integer=w187:i32)
        n52 = call <vilib>:"Mean PtByPt.vi"("x"=w184, "sample length"=w187) -> ("mean"=w186:dbl)  [unwired: 1 in, 2 out]
        n53 = formula code="ScaledOut = ((Vin-Offset)*Slope);\nVout=Vin;"("Vin"=w186, "Slope"=w183, "Offset"=w182) -> ("ScaledOut"=w181:dbl, "Vout"=w180:dbl)
      }
      frame 12 {
        # "13    CH12\t\tPins  56/57\t  P4 Fuel 0-1000"
        # "Ind# USB#1"
        n54 = To Long Integer(number=w193) -> (32bit integer=w195:i32)
        n55 = call <vilib>:"Mean PtByPt.vi"("x"=w192, "sample length"=w195) -> ("mean"=w194:dbl)  [unwired: 1 in, 2 out]
        n56 = formula code="ScaledOut = ((Vin-Offset)*Slope);\nVout=Vin;"("Vin"=w194, "Slope"=w191, "Offset"=w190) -> ("ScaledOut"=w189:dbl, "Vout"=w188:dbl)
      }
      frame 13 {
        # "14    CH13\t\tPins  58/59\t  P3 Fuel 0-1000"
        # "Ind# USB#1"
        n57 = To Long Integer(number=w201) -> (32bit integer=w203:i32)
        n58 = call <vilib>:"Mean PtByPt.vi"("x"=w200, "sample length"=w203) -> ("mean"=w202:dbl)  [unwired: 1 in, 2 out]
        n59 = formula code="ScaledOut = ((Vin-Offset)*Slope);\nVout=Vin;"("Vin"=w202, "Slope"=w199, "Offset"=w198) -> ("ScaledOut"=w197:dbl, "Vout"=w196:dbl)
      }
      frame 14 {
        # "15    CH14\t\tPins  61/62 \t P2 Fuel 0-1000"
        # "Ind# USB#1"
        n60 = To Long Integer(number=w209) -> (32bit integer=w211:i32)
        n61 = call <vilib>:"Mean PtByPt.vi"("x"=w208, "sample length"=w211) -> ("mean"=w210:dbl)  [unwired: 1 in, 2 out]
        n62 = formula code="ScaledOut = ((Vin-Offset)*Slope);\nVout=Vin;"("Vin"=w210, "Slope"=w207, "Offset"=w206) -> ("ScaledOut"=w205:dbl, "Vout"=w204:dbl)
      }
      frame 15 {
        # "16    CH15\t\tPins  63/64 \t P1 Fuel 0-1500"
        # "Ind# USB#1"
        n63 = To Long Integer(number=w217) -> (32bit integer=w219:i32)
        n64 = call <vilib>:"Mean PtByPt.vi"("x"=w216, "sample length"=w219) -> ("mean"=w218:dbl)  [unwired: 1 in, 2 out]
        n65 = formula code="ScaledOut = ((Vin-Offset)*Slope);\nVout=Vin;"("Vin"=w218, "Slope"=w215, "Offset"=w214) -> ("ScaledOut"=w213:dbl, "Vout"=w212:dbl)
      }
      frame 16 {
        # "17    CH16\t\tPins  15/16\t DP1 Fuel 0-100"
        # "Ind# USB#1"
        n66 = To Long Integer(number=w225) -> (32bit integer=w227:i32)
        n67 = call <vilib>:"Mean PtByPt.vi"("x"=w224, "sample length"=w227) -> ("mean"=w226:dbl)  [unwired: 1 in, 2 out]
        n68 = formula code="ScaledOut = ((Vin-Offset)*Slope);\nVout=Vin;"("Vin"=w226, "Slope"=w223, "Offset"=w222) -> ("ScaledOut"=w221:dbl, "Vout"=w220:dbl)
      }
      frame 17 {
        # "18    CH17\t\tPins  17/18\t DP2 Fuel 0-100"
        # "Ind# USB#2"
        n69 = To Long Integer(number=w233) -> (32bit integer=w235:i32)
        n70 = call <vilib>:"Mean PtByPt.vi"("x"=w232, "sample length"=w235) -> ("mean"=w234:dbl)  [unwired: 1 in, 2 out]
        n71 = formula code="ScaledOut = ((Vin-Offset)*Slope);\nVout=Vin;"("Vin"=w234, "Slope"=w231, "Offset"=w230) -> ("ScaledOut"=w229:dbl, "Vout"=w228:dbl)
      }
      frame 18 {
        # "19    CH18\t\tPins  19/20  DP3 Fuel 0-500"
        # "Ind# USB#2"
        n72 = To Long Integer(number=w241) -> (32bit integer=w243:i32)
        n73 = call <vilib>:"Mean PtByPt.vi"("x"=w240, "sample length"=w243) -> ("mean"=w242:dbl)  [unwired: 1 in, 2 out]
        n74 = formula code="ScaledOut = ((Vin-Offset)*Slope);\nVout=Vin;"("Vin"=w242, "Slope"=w239, "Offset"=w238) -> ("ScaledOut"=w237:dbl, "Vout"=w236:dbl)
      }
      frame 19 {
        # "20    CH19\t Pins  21/22\t Lube Level 0-2"
        # "Ind# USB#2"
        n75 = To Long Integer(number=w249) -> (32bit integer=w251:i32)
        n76 = call <vilib>:"Mean PtByPt.vi"("x"=w248, "sample length"=w251) -> ("mean"=w250:dbl)  [unwired: 1 in, 2 out]
        n77 = formula code="ScaledOut = ((Vin-Offset)*Slope);\nVout=Vin;"("Vin"=w250, "Slope"=w247, "Offset"=w246) -> ("ScaledOut"=w245:dbl, "Vout"=w244:dbl)
      }
      frame 20 {
        # "21    CH20\t\tPins  24/25\t Fuel Level 0-2"
        # "Ind# USB#2"
        n78 = To Long Integer(number=w257) -> (32bit integer=w259:i32)
        n79 = call <vilib>:"Mean PtByPt.vi"("x"=w256, "sample length"=w259) -> ("mean"=w258:dbl)  [unwired: 1 in, 2 out]
        n80 = formula code="ScaledOut = ((Vin-Offset)*Slope);\nVout=Vin;"("Vin"=w258, "Slope"=w255, "Offset"=w254) -> ("ScaledOut"=w253:dbl, "Vout"=w252:dbl)
      }
      frame 21 {
        # "22    CH21\t\tPins  26/27\tTM1 Volts"
        # "Ind# USB#2"
        n81 = To Long Integer(number=w265) -> (32bit integer=w267:i32)
        n82 = call <vilib>:"Mean PtByPt.vi"("x"=w264, "sample length"=w267) -> ("mean"=w266:dbl)  [unwired: 1 in, 2 out]
        n83 = formula code="ScaledOut = ((Vin-Offset)*Slope);\nVout=Vin;"("Vin"=w266, "Slope"=w263, "Offset"=w262) -> ("ScaledOut"=w260:dbl, "Vout"=w261:dbl)
      }
      frame 22 {
        # "23    CH22\t Pins  29/30  Fuel Res Temp       TC1"
        # "Ind# USB#2"
        n84 = To Long Integer(number=w273) -> (32bit integer=w275:i32)
        n85 = call <vilib>:"Mean PtByPt.vi"("x"=w272, "sample length"=w275) -> ("mean"=w274:dbl)  [unwired: 1 in, 2 out]
        n86 = formula code="ScaledOut = ((Vin-Offset)*Slope);\nVout=Vin;"("Vin"=w274, "Slope"=w271, "Offset"=w270) -> ("ScaledOut"=w269:dbl, "Vout"=w268:dbl)
      }
      frame 23 {
        # "24    CH23\t\tPins  31/32\t Fuel Temp (Panel)  TC2"
        # "Ind# USB#2"
        n87 = To Long Integer(number=w281) -> (32bit integer=w283:i32)
        n88 = call <vilib>:"Mean PtByPt.vi"("x"=w280, "sample length"=w283) -> ("mean"=w282:dbl)  [unwired: 1 in, 2 out]
        n89 = formula code="ScaledOut = ((Vin-Offset)*Slope);\nVout=Vin;"("Vin"=w282, "Slope"=w279, "Offset"=w278) -> ("ScaledOut"=w277:dbl, "Vout"=w276:dbl)
      }
      frame 24 {
        # "25    CH24\t\tPins \t47/48\t Lube Res Temp     TC3"
        # "Ind# USB#2"
        n90 = To Long Integer(number=w289) -> (32bit integer=w291:i32)
        n91 = call <vilib>:"Mean PtByPt.vi"("x"=w288, "sample length"=w291) -> ("mean"=w290:dbl)  [unwired: 1 in, 2 out]
        n92 = formula code="ScaledOut = ((Vin-Offset)*Slope);\nVout=Vin;"("Vin"=w290, "Slope"=w287, "Offset"=w286) -> ("ScaledOut"=w285:dbl, "Vout"=w284:dbl)
      }
      frame 25 {
        # "26    CH25\t\tPins  49/50\t Lub  Temp (Panel) TC4"
        # "Ind# USB#2"
        n93 = To Long Integer(number=w297) -> (32bit integer=w299:i32)
        n94 = call <vilib>:"Mean PtByPt.vi"("x"=w296, "sample length"=w299) -> ("mean"=w298:dbl)  [unwired: 1 in, 2 out]
        n95 = formula code="ScaledOut = ((Vin-Offset)*Slope);\nVout=Vin;"("Vin"=w298, "Slope"=w295, "Offset"=w294) -> ("ScaledOut"=w293:dbl, "Vout"=w292:dbl)
      }
      frame 26 {
        # "27    CH26\t\tPins  51/52\t RTD"
        # "Ind# USB#2"
        n96 = To Long Integer(number=w305) -> (32bit integer=w307:i32)
        n97 = call <vilib>:"Mean PtByPt.vi"("x"=w304, "sample length"=w307) -> ("mean"=w306:dbl)  [unwired: 1 in, 2 out]
        n98 = formula code="ScaledOut = ((Vin-Offset)*Slope);\nVout=Vin;"("Vin"=w306, "Slope"=w303, "Offset"=w302) -> ("ScaledOut"=w301:dbl, "Vout"=w300:dbl)
      }
      frame 27 {
        # "28    CH27\t\tPins  53/54\t TM1 Amps"
        # "Ind# USB#2"
        n99 = To Long Integer(number=w313) -> (32bit integer=w315:i32)
        n100 = call <vilib>:"Mean PtByPt.vi"("x"=w312, "sample length"=w315) -> ("mean"=w314:dbl)  [unwired: 1 in, 2 out]
        n101 = formula code="ScaledOut = ((Vin-Offset)*Slope);\nVout=Vin;"("Vin"=w314, "Slope"=w311, "Offset"=w310) -> ("ScaledOut"=w308:dbl, "Vout"=w309:dbl)
      }
      frame 28 {
        # "29    CH28\t\tPins  56/57\t TM2 Volts"
        # "Ind# USB#2"
        n102 = To Long Integer(number=w321) -> (32bit integer=w323:i32)
        n103 = call <vilib>:"Mean PtByPt.vi"("x"=w320, "sample length"=w323) -> ("mean"=w322:dbl)  [unwired: 1 in, 2 out]
        n104 = formula code="ScaledOut = ((Vin-Offset)*Slope);\nVout=Vin;"("Vin"=w322, "Slope"=w319, "Offset"=w318) -> ("ScaledOut"=w316:dbl, "Vout"=w317:dbl)
      }
      frame 29 {
        # "30    CH29\t\tPins  58/59\t TM2 Amps"
        # "Ind# USB#2"
        n105 = To Long Integer(number=w329) -> (32bit integer=w331:i32)
        n106 = call <vilib>:"Mean PtByPt.vi"("x"=w328, "sample length"=w331) -> ("mean"=w330:dbl)  [unwired: 1 in, 2 out]
        n107 = formula code="ScaledOut = ((Vin-Offset)*Slope);\nVout=Vin;"("Vin"=w330, "Slope"=w327, "Offset"=w326) -> ("ScaledOut"=w324:dbl, "Vout"=w325:dbl)
      }
      frame 30 {
        # "31    CH30\t\tPins  61/62  Solenoid Power Volts"
        # "Ind# USB#2"
        n108 = To Long Integer(number=w337) -> (32bit integer=w339:i32)
        n109 = call <vilib>:"Mean PtByPt.vi"("x"=w336, "sample length"=w339) -> ("mean"=w338:dbl)  [unwired: 1 in, 2 out]
        n110 = formula code="ScaledOut = ((Vin-Offset)*Slope);\nVout=Vin;"("Vin"=w338, "Slope"=w335, "Offset"=w334) -> ("ScaledOut"=w332:dbl, "Vout"=w333:dbl)
      }
      frame 31 {
        # "32    CH31\t\tPins  63/64  Solenoid Power Amps"
        # "Ind# USB#2"
        n111 = To Long Integer(number=w345) -> (32bit integer=w347:i32)
        n112 = call <vilib>:"Mean PtByPt.vi"("x"=w344, "sample length"=w347) -> ("mean"=w346:dbl)  [unwired: 1 in, 2 out]
        n113 = formula code="ScaledOut = ((Vin-Offset)*Slope);\nVout=Vin;"("Vin"=w346, "Slope"=w343, "Offset"=w342) -> ("ScaledOut"=w340:dbl, "Vout"=w341:dbl)
      }
    }
  }
  "ScaledOut" <- w10
  n114 = Number To Fractional String(number=w19, precision (6)=i16 6) -> (F-format string=→"Vout":string[])  [unwired: 2 out]
  n115 = Number To Fractional String(number=w10, precision (6)=i16 6) -> (F-format string=→"ScaledOut":string[])  [unwired: 2 out]
  "Allow Zero?" <- "Allow Zero?"
  "Offset Data" <- "Offset Data"
  "error out" <- "error in"
